vi "Launch Progress Bar.vi"(8 "error in (no error)":errorcluster) -> (0 "error out":errorcluster)   [LabVIEW 2013, in "Progress Bar.lvlib"]
uses:
  Progress Bar.lvlib
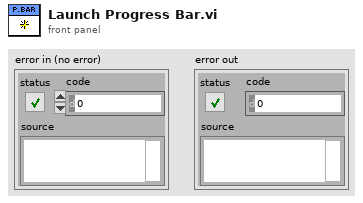
[diagram p1: front panel]
types:
  T1 = typedef "Rendezvous RefNum" = refnum<k1>
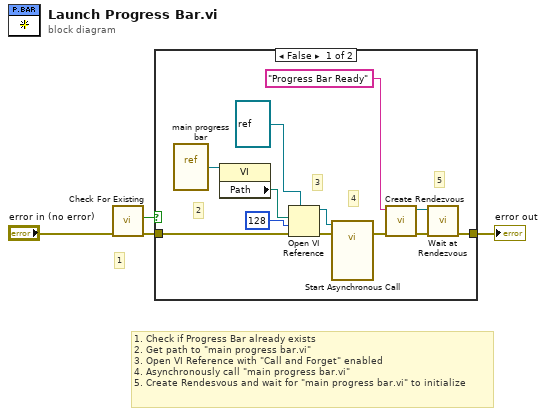
[diagram p0: block diagram]
diagram:
  # "1"
  # "1. Check if Progress Bar already exists\n2. Get path to \"main progress bar.vi\" \n3. Open VI Reference with \"Call and Forget\" enabled\n4. Asynchronously call \"main progress bar.vi\"\n5. Create Rendesvous and wait for \"main progress bar.vi\" to initialize"
  n1 = call "Check For Existing.vi"("error in (no error)"="error in (no error)") -> ("error out"=w1:errorcluster, "Exists?"=w3:bool)  [unwired: 9 in]
  n2 = case shown="False" w3 {
    tunnel: w1 -> [w13 w17]
    tunnel: [w5 w17] -> w4
    frame False {
      # "5"
      # "4"
      # "3"
      # "2"
      n3 = vi-ref "main progress bar.vi"() -> (w12:refnum<vi>)
      n4 = property class="VI"(reference=w12) -> ("Path"=w11:path)  [unwired: 1 in, 2 out]
      n5 = Open VI Reference(type specifier VI Refnum (for type only)=refnum<vi> refnum, vi path=w11, options=128, error in (no error)=w13) -> (vi reference=w14:refnum<vi>, error out=w10:errorcluster)  [unwired: 2 in]
      n6 = call-by-ref "Start Asynchronous Call"(reference=w14, error in=w10) -> (error out=w6:errorcluster)  [unwired: 11 in, 2 out]
      n7 = call <vilib>:"Create Rendezvous.vi"("error in (no error)"=w6, "name (unnamed)"="Progress Bar Ready") -> ("error out"=w8:errorcluster, "rendezvous"=w7:T1)  [unwired: 3 in, 1 out]
      n8 = call <vilib>:"Wait at Rendezvous.vi"("error in (no error)"=w8, "rendezvous"=w7) -> ("error out"=w5:errorcluster)  [unwired: 3 in, 2 out]
    }
    frame True {
    }
  }
  "error out" <- w4
